vi "Write U64 Direct Dispatch.vi"(8 "error in (no error)":errorcluster, 9 "Timeout (ms)":i32, 10 "Data":u64, 11 "CIFTag in":refnum<class "CIFChannels.lvclass">) -> (0 "error out":errorcluster, 1 "timed out?":bool, 3 "CIFTag out":refnum<class "CIF_NIChn_U64.lvclass">)   [LabVIEW 2021, in "CIF_NIChn_U64.lvclass"]
uses:
  CIF_NIChn_U64.lvclass
  D:/dev/CIF-LVCore/src/Channels/CIF_NIChn/NIChn/CIF_NIChnl.lvclass
  CIFChannels/CIFChannels.lvclass
  NIChn/CIF_NIChn.lvclass/CIF_NIChn.ctl
  CIF_NIChn_U64.lvclass/CIF_NIChn_U64.ctl
  e6e5dc56-0fe0-434b-816e-55c2e61471c2.vi
  e6e5dc56-0fe0-434b-816e-55c2e61471c2.vi/4bc1c15b-36ab-481f-b8dd-c64075ce723a.vi
  e6e5dc56-0fe0-434b-816e-55c2e61471c2.vi/d83cb72b-7713-41fc-a3d1-682de79cf574.vi
  <vilib>/CIFChannels/SubVIs/Get dll Path.vi
  NIChn/CIF_NIChn.lvclass
  D:/dev/CIF-LVCore/src/Channels/CIF_NIChn/NIChn/CIF_NIChn.lvclass
  D:/dev/CIF-LVCore/src/Channels/CIFChannels/CIFChannels.lvclass
  D:/dev/CIF-LVCore/src/Channels/CIF_NIChn/U64/CIF_NIChn_U64.lvclass
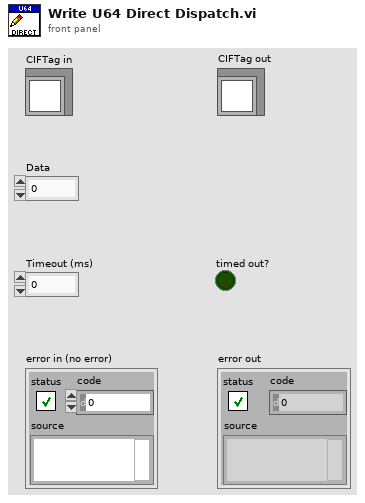
[diagram p1: front panel]
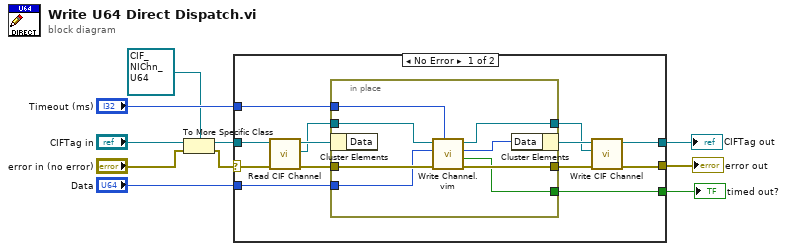
[diagram p0: block diagram]
diagram:
  n1 = To More Specific Class(target class=refnum<class "CIF_NIChn_U64.lvclass"> refnum ("CIFTag in"), reference="CIFTag in", error in="error in (no error)") -> (specific class reference=w3:refnum<class "CIF_NIChn_U64.lvclass">, error out=w1:errorcluster)
  n2 = case shown="No Error" w1 {
    selector: w1 -> [w20 w33]
    tunnel: [w14 w33] -> w10
    tunnel: [w16 w32] -> w9
    tunnel: w3 -> [w21 w32]
    tunnel: "Data" -> [w23 _]
    tunnel: [w22 _] -> w7
    tunnel: "Timeout (ms)" -> [w11 _]
    frame No Error {
      n3 = call "Read CIF Channel.vi"("error in (no error)"=w20, "CIFTag in"=w21) -> ("error out"=w18:errorcluster, "CIF Channel"=w13:refnum<k21>, "CIFTag out"=w19:refnum<class "CIF_NIChn_U64.lvclass">)  [unwired: 7 in]
      n4 = in-place {
        in-place-border: w18 -> [w31]
        in-place-border: [w30] -> w15
        in-place-border: w23 -> [w28]
        in-place-border: [w29] -> w22
        in-place-border: w13 -> [w26]
        in-place-border: [w25] -> w12
        in-place-border: w11 -> [w24]
        n5 = in-place-cluster #1(w19) -> ()  [unwired: 1 out]
        n6 = call "Write Channel.vim"("Timeout (ms)"=w24, "error in"=w31, "Data in"=w28, "CIF Channel in"=w26) -> ("error out"=w30:errorcluster, "Timed out?"=w29:bool, "Data out"=w27:u64, "CIF Channel out"=w25:refnum<k21>)  [unwired: 4 in]
        n7 = in-place-cluster #1("Data"=w27) -> (w17:refnum<class "CIF_NIChn_U64.lvclass">)
      }
      n8 = call "Write CIF Channel.vi"("error in (no error)"=w15, "CIF Channel"=w12, "CIFTag in"=w17) -> ("error out"=w14:errorcluster, "CIFTag out"=w16:refnum<class "CIF_NIChn_U64.lvclass">)  [unwired: 7 in]
    }
    frame Error {
    }
  }
  "error out" <- w10
  "CIFTag out" <- w9
  "timed out?" <- w7
